vi "LVProjectShortcut_Item_Interface.vi"() -> (3 "InterfaceTable":T1)   [LabVIEW 2017, in "LVProject Shortcut.lvlib"]
uses:
  <resource>/Framework/Providers/API/Item_Interface.ctl
  LVProject Shortcut.lvlib
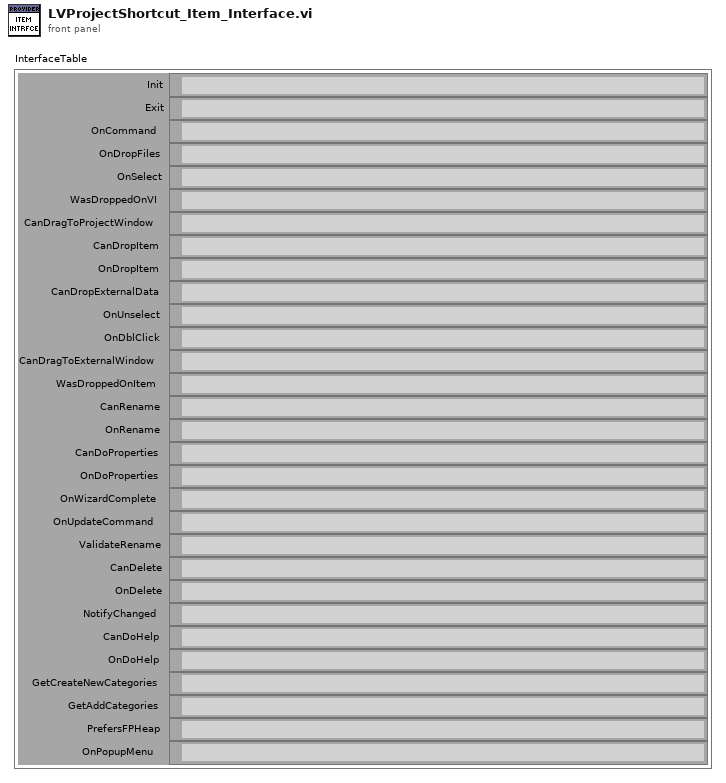
[diagram p1: front panel]
types:
  T1 = typedef "Item_Interface.ctl" = cluster{"Init":path, "Exit":path, "OnCommand":path, "OnDropFiles":path, "OnSelect":path, "WasDroppedOnVI":path, "CanDragToProjectWindow":path, "CanDropItem":path, "OnDropItem":path, "CanDropExternalData":path, "OnUnselect":path, "OnDblClick":path, "CanDragToExternalWindow":path, "WasDroppedOnItem":path, "CanRename":path, "OnRename":path, "CanDoProperties":path, "OnDoProperties":path, "OnWizardComplete":path, "OnUpdateCommand":path, "ValidateRename":path, "CanDelete":path, "OnDelete":path, "NotifyChanged":path, "CanDoHelp":path, "OnDoHelp":path, "GetCreateNewCategories":path, "GetAddCategories":path, "PrefersFPHeap":path, "OnPopupMenu":path}
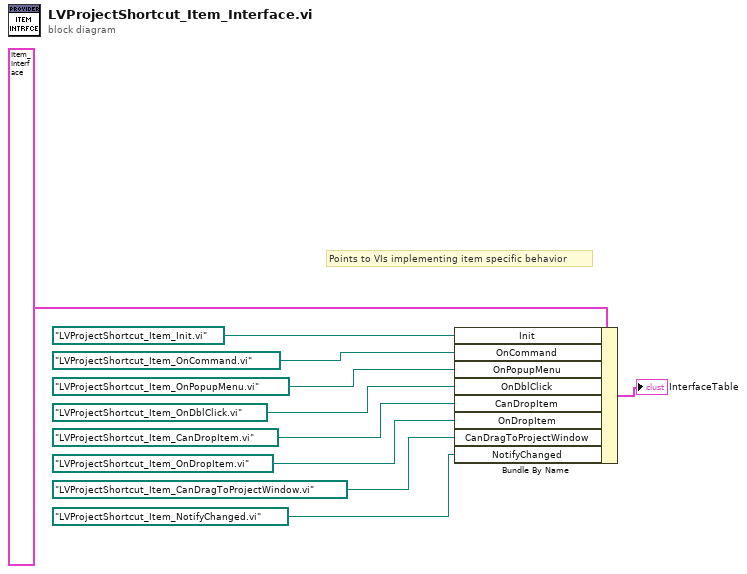
[diagram p0: block diagram]
diagram:
  # "Points to VIs implementing item specific behavior"
  n1 = Bundle By Name(cluster=T1 {"Init"=path "", "Exit"=path "", "OnCommand"=path "", "OnDropFiles"=path "", "OnSelect"=path "", "WasDroppedOnVI"=path "", "CanDragToProjectWindow"=path "", "CanDropItem"=path "", "OnDropItem"=path "", "CanDropExternalData"=path "", "OnUnselect"=path "", "OnDblClick"=path "", "CanDragToExternalWindow"=path "", "WasDroppedOnItem"=path "", "CanRename"=path "", "OnRename"=path "", "CanDoProperties"=path "", "OnDoProperties"=path "", "OnWizardComplete"=path "", "OnUpdateCommand"=path "", "ValidateRename"=path "", "CanDelete"=path "", "OnDelete"=path "", "NotifyChanged"=path "", "CanDoHelp"=path "", "OnDoHelp"=path "", "GetCreateNewCategories"=path "", "GetAddCategories"=path "", "PrefersFPHeap"=path "", "OnPopupMenu"=path ""} ("InterfaceTable"), "Init"=path "LVProjectShortcut_Item_Init.vi", "OnCommand"=path "LVProjectShortcut_Item_OnCommand.vi", "OnPopupMenu"=path "LVProjectShortcut_Item_OnPopupMenu.vi", "OnDblClick"=path "LVProjectShortcut_Item_OnDblClick.vi", "CanDropItem"=path "LVProjectShortcut_Item_CanDropItem.vi", "OnDropItem"=path "LVProjectShortcut_Item_OnDropItem.vi", "CanDragToProjectWindow"=path "LVProjectShortcut_Item_CanDragToProjectWindow.vi", "NotifyChanged"=path "LVProjectShortcut_Item_NotifyChanged.vi" ("CanDragToProjectWindow")) -> (→"InterfaceTable":T1)
